vi "Start Capture.vi"(4 "Error":string) -> (0 "Error":string, 1 "Height":i32, 2 "Width":i32)   [LabVIEW 2011, in "labvvis.lvlib"]
doc: "Returns the width and height of a LabVVIS image."
uses:
  <userlib>/labvvis/labvvis.lvlib
  labvvis.framework
panel:
  in  "Height":i32
  in  "Width":i32
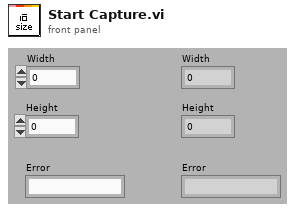
[diagram p1: front panel]
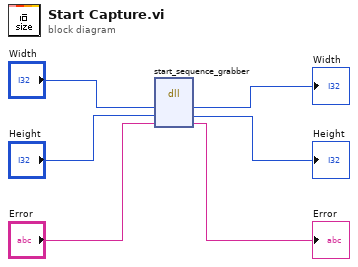
[diagram p0: block diagram]
diagram:
  n1 = dll-call lib="labvvis.framework" fn="start_sequence_grabber"("width"="Width", "height"="Height", "error"="Error") -> ("width"=→"Width":i32, "height"=→"Height":i32, "error"=→"Error":string)  [unwired: 4 in, 2 out]
